vi "LDA_BSA_Comms_F600.vi"(2 "LDA Channels":T1[](array[typedef]) {"Sync Delay (s)" format="%.2g"; "Req Sampling Rate Hz" min=1.0; "Shifted mW" format="%.1g"; "Unshifted mW" format="%.1g"; "Centre Velocity (m/s)" format="%.2g"; "Velocity Range (m/s)" format="%.2g"; "Focal Length (mm)" format="%.1f"; "Beam Separation (mm)" format="%.1f"; "Optics Conversion Factor" format="%.3g"; "High voltage" min=0 max=2040 step=8; "Signal gain (dB)" min=0 max=30 step=1; "Min Velocity" format="%.2g"; "Max Velocity" format="%.2g"; "Wavelength (nm)" format="%.1f"}, 3 "BSACtrl.IBSA F600":refnum<k7>) -> (0 "error out":errorcluster, 1 "LDA Raw Data":cluster{dbl[][]}[](array[cluster]))   [LabVIEW 2021]
uses:
  LDA_Channel.ctl
  Globals/Meas_global.vi
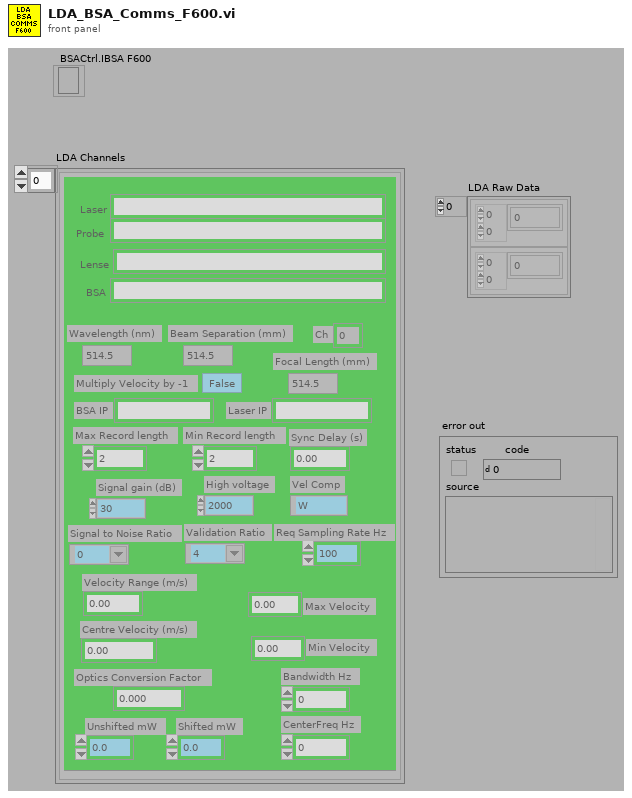
[diagram p1: front panel]
types:
  T1 = typedef "LDA_Channel.ctl" = cluster{"Wavelength (nm)":dbl, "Vel Comp":string, "Max Velocity":dbl, "Min Velocity":dbl, "Max Record length":u16, "Signal gain (dB)":i16, "High voltage":i16, "Optics Conversion Factor":dbl, "Min Record length":u16, "Multiply Velocity by -1":bool, "Signal to Noise Ratio":string, "Validation Ratio":string, "Probe":string, "Laser":string, "BSA":string, "Lense":string, "Beam Separation (mm)":dbl, "Focal Length (mm)":dbl, "COLOUR":u32, "BSA IP":string, "Velocity Range (m/s)":dbl, "Centre Velocity (m/s)":dbl, "Unshifted mW":dbl, "Shifted mW":dbl, "Bandwidth Hz":dbl, "Req Sampling Rate Hz":dbl, "Ch":i32, "CenterFreq Hz":dbl, "Laser IP":string, "Sync Delay (s)":dbl}
  T2 = typedef "Analysis_info_cluster.ctl" = cluster{"Colour":u32, "Inst type":T3, "Inst name":string, "Symbol":string, "Code name":string, "Extra Info":string, "Inst Array":T4, "Extra Titles":string[], "Extra Values":string[], "U":dbl, "u^2":dbl, "u^3":dbl, "u^4":dbl, "Skew_u":dbl, "Kurt_u":dbl, "Sd Error in Mean":dbl, "% u'/U":dbl, "X":dbl, "Y":dbl, "Z":dbl, "Timescale integral Estimate":dbl, "Sd Error in Variance":dbl, "Calib File":path, "Calib Constants":dbl[], "Output Position":bool, "Stats":enum16{"None", "Basic", "Full"}, "Av Sampling Rate":dbl, "Av No of Samples":dbl, "Total Meas Time (s)":dbl, "ADAM Ch Name":string, "Max value":dbl, "Min value":dbl, "Req Sample Rate Hz":dbl, "Sync Delay Time (s)":dbl, "Ch No":i16, "Device":string, "Use Latest Calib":bool, "Port":string, "Metadata Ch Names":string[], "Metadata Ch Values":string[], "Label":string}
  T3 = typedef "Inst_type.ctl" = enum16{"Raw voltage", "Raw with zero offsetting", "Propeller anemometer", "Pressure Transducer", "Pitot-static tube", "Hot wire", "Cross wire 1", "Cross wire 2", "Generic Linear", "Generic Polynomial", "Generic BackPoly", "Fast FID", "Thermocouple", "Cold wire", "Pulsed Wire", "LDA Vel", "LDA Tran time", "LDA Arr time", "Microphone"}
  T4 = typedef "Instrument_Array.ctl" = enum16{"PWA", "LDA", "Analogue"}
  T5 = typedef "Trigger_Mode.ctl" = enum16{"Free Running", "Start on Trigger", "Trigger Every Block", "Trigger Every Sample"}
  T6 = typedef "Rendezvous RefNum" = refnum<k1>
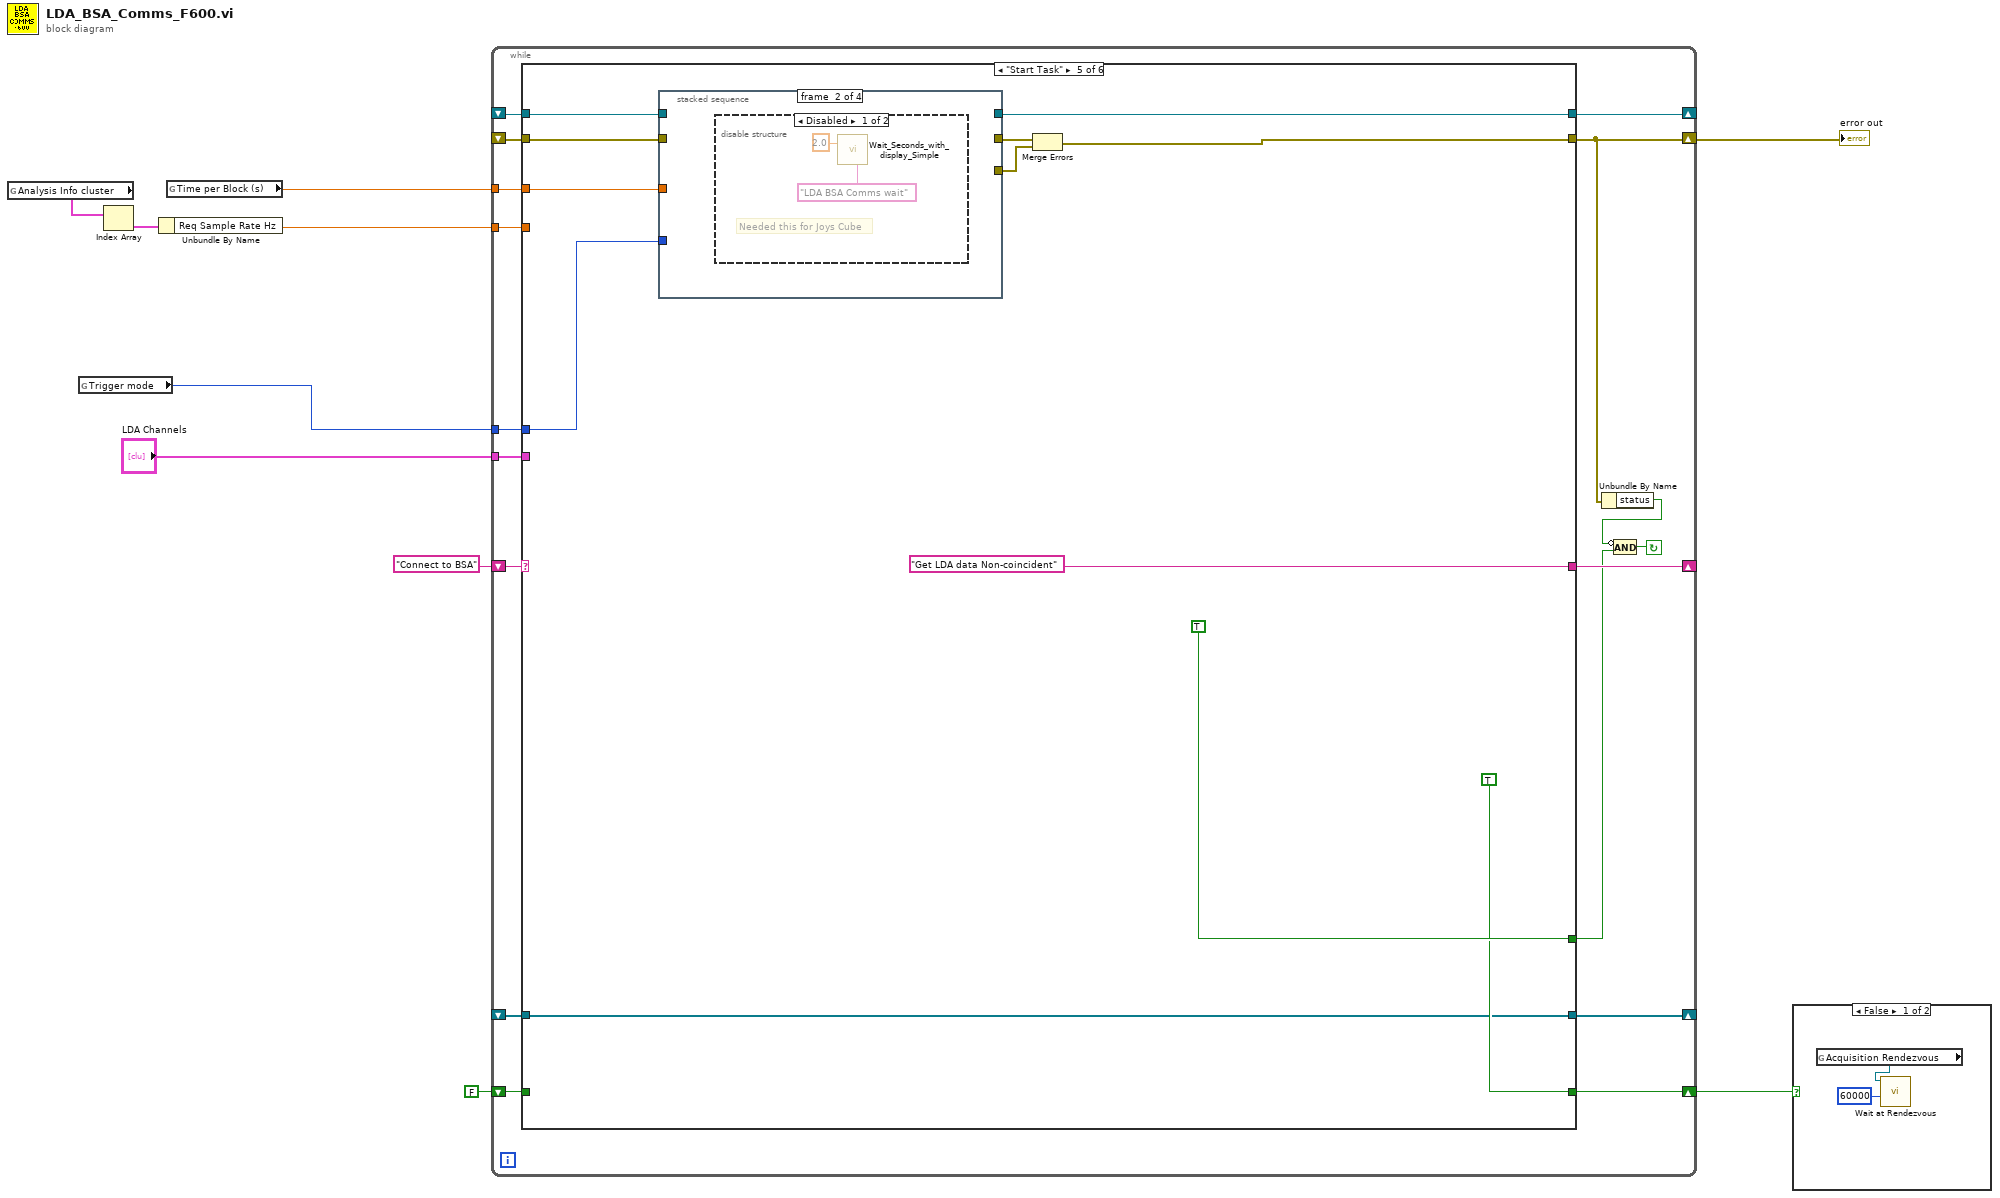
[diagram p0: block diagram]
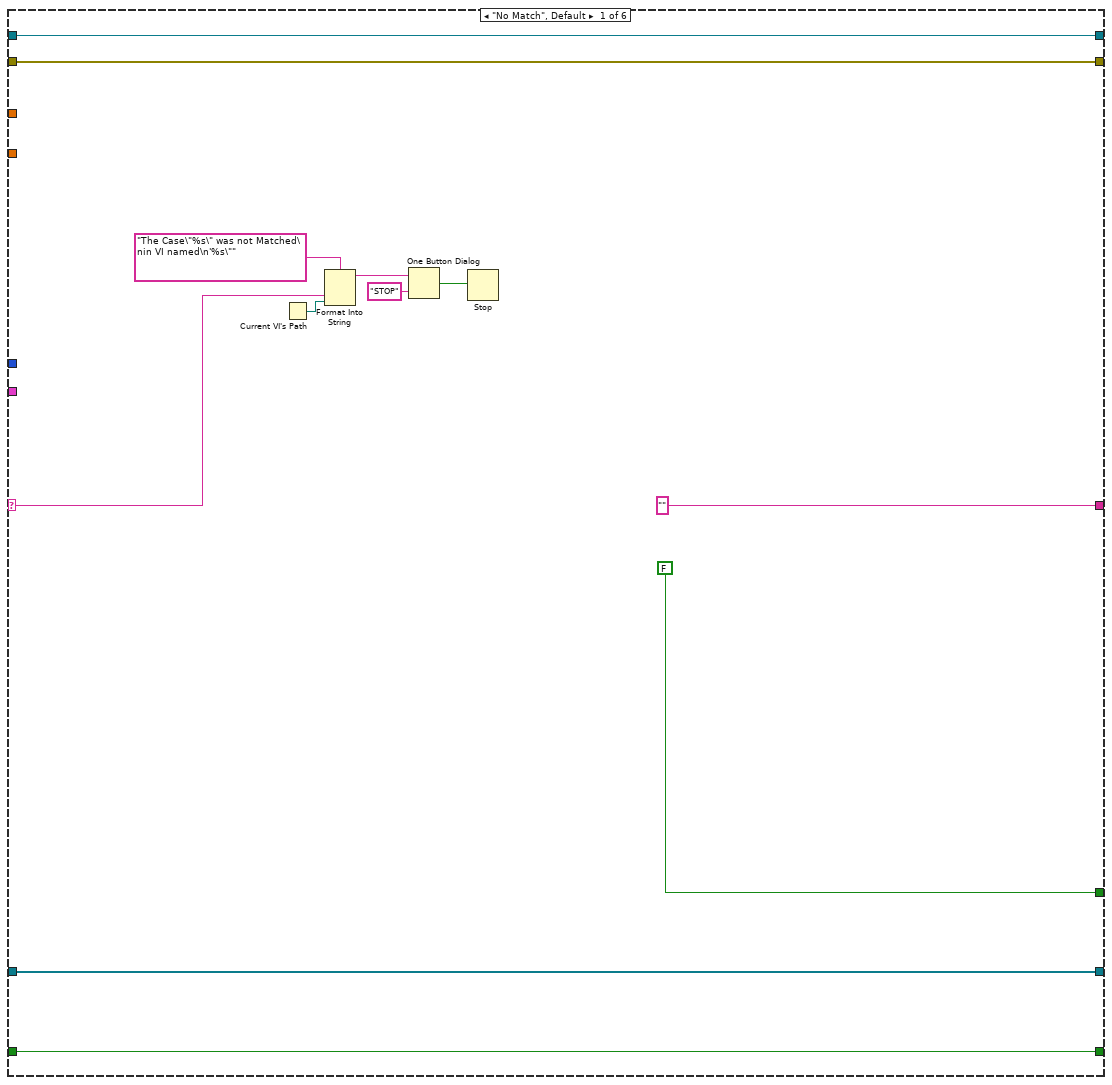
[diagram p2: hidden frame]
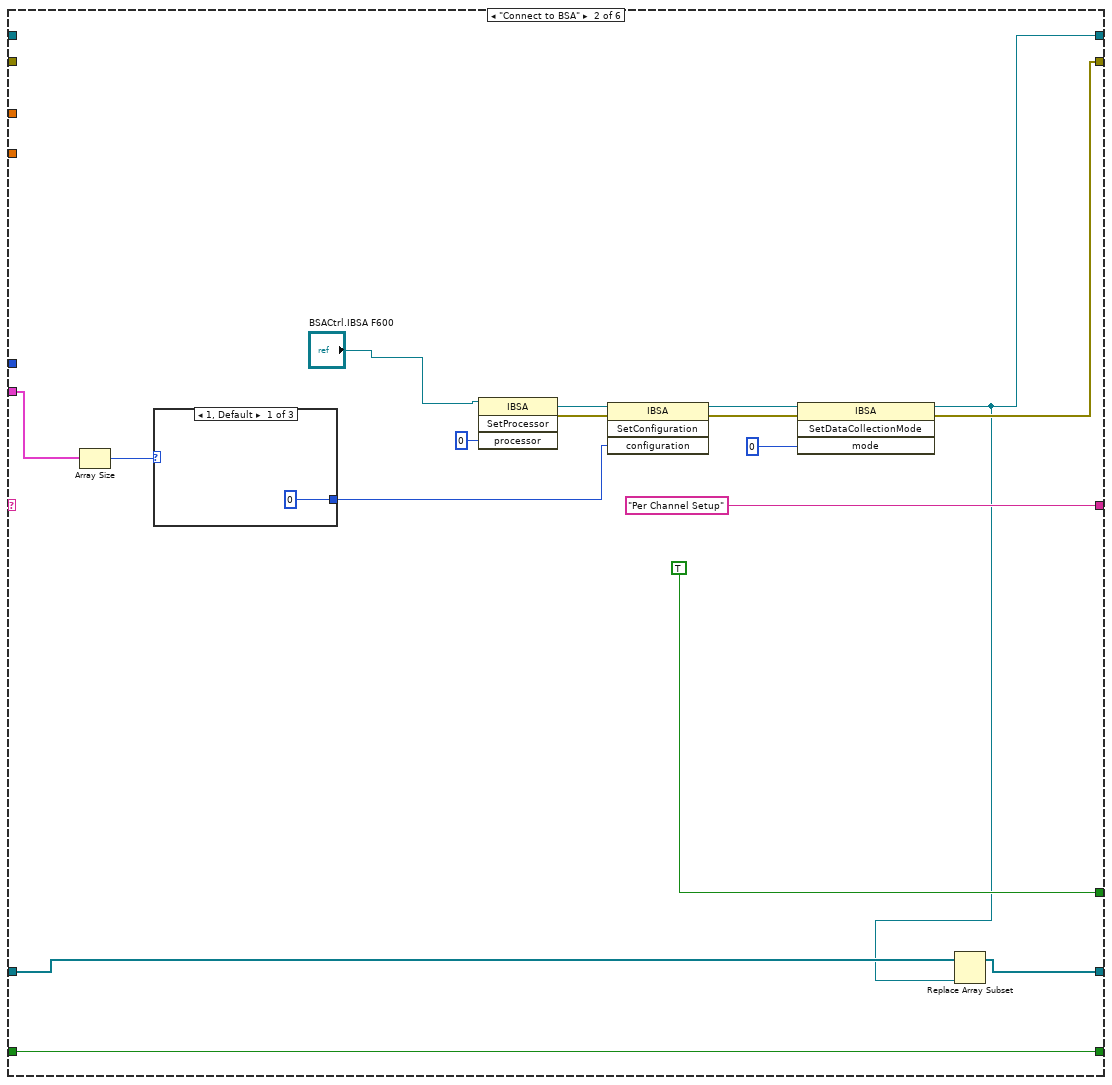
[diagram p3: hidden frame]
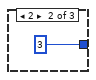
[diagram p4: hidden frame]
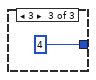
[diagram p5: hidden frame]
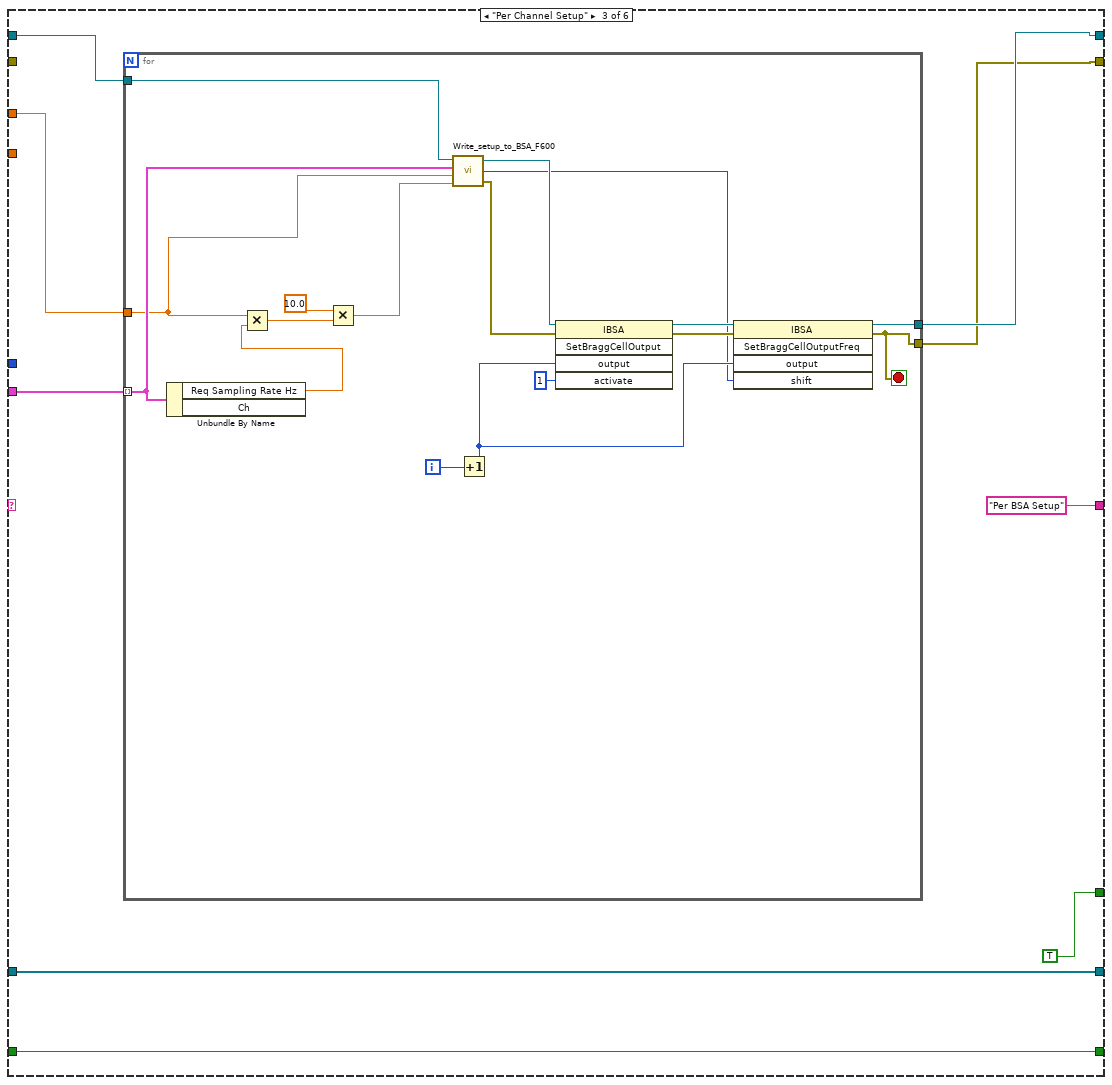
[diagram p6: hidden frame]
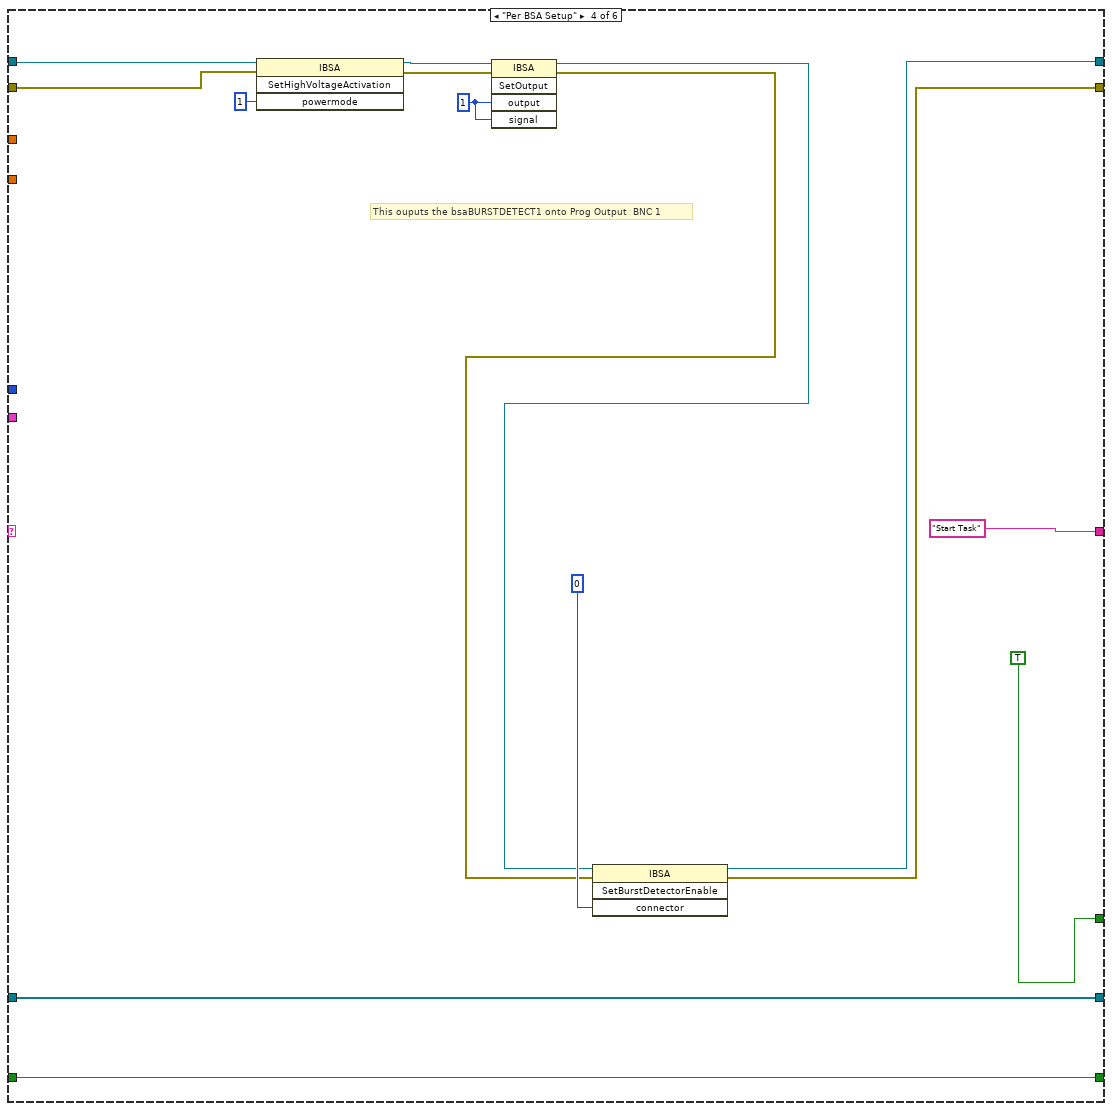
[diagram p7: hidden frame]
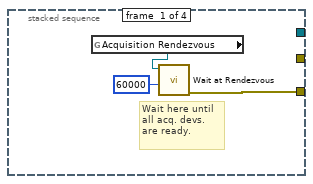
[diagram p8: hidden frame]
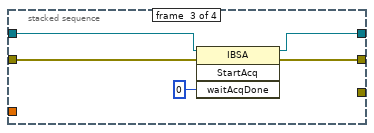
[diagram p10: hidden frame]
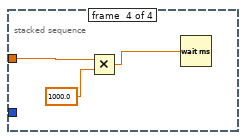
[diagram p11: hidden frame]
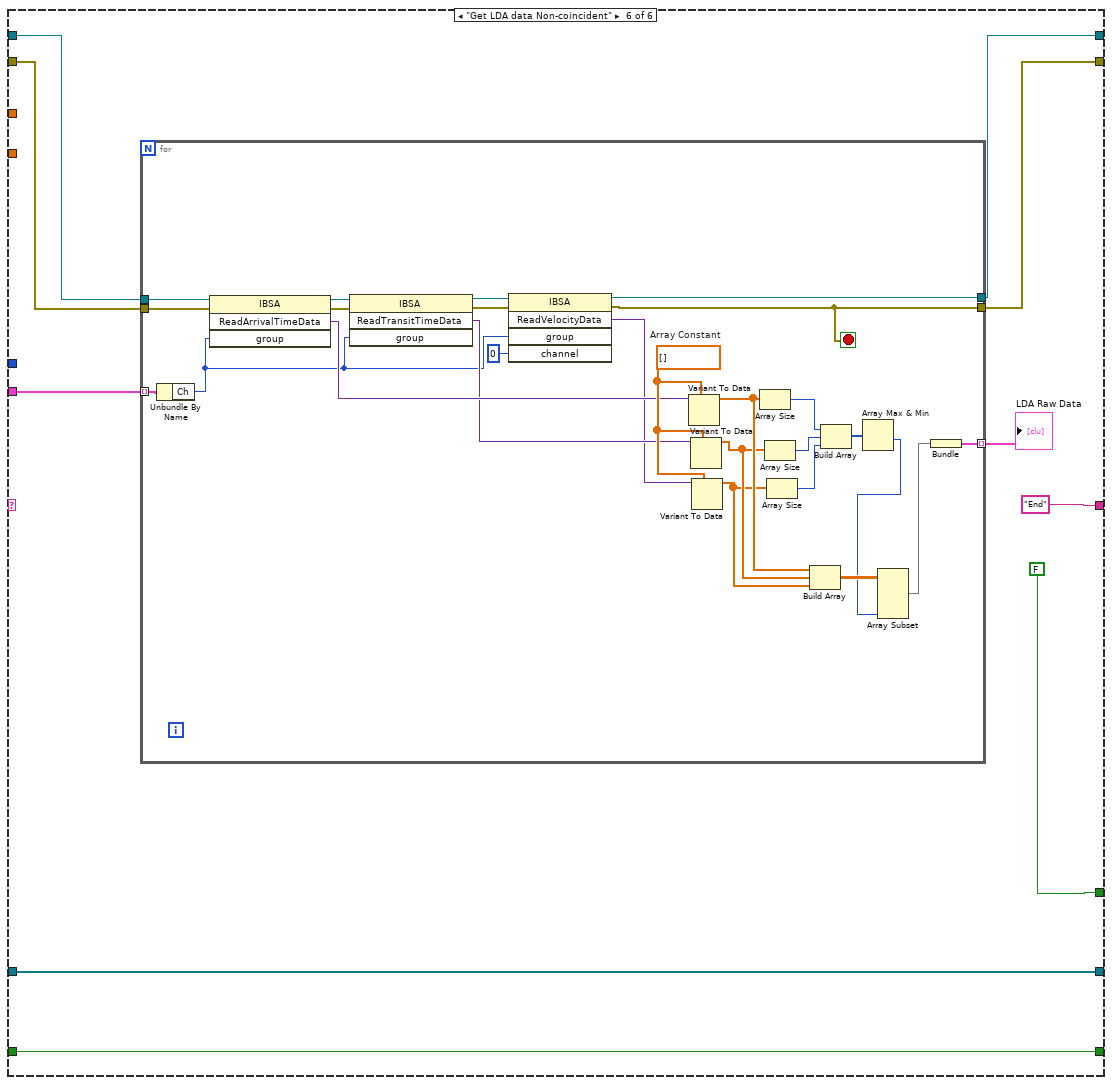
[diagram p12: hidden frame]
diagram:
  n1 = global read "Meas_global.vi" "Analysis Info cluster"() -> (w10:T2[])
  n2 = global read "Meas_global.vi" "Trigger mode"() -> (w6:T5)
  n3 = Index Array(array=w10) -> (element=w9:T2)  [unwired: 1 in]
  n4 = Unbundle By Name(w9) -> ("Req Sample Rate Hz"=w8:dbl)
  n5 = global read "Meas_global.vi" "Time per Block (s)"() -> (w7:dbl)
  n6 = while {
    shift-left: "Connect to BSA" -> [w26]
    shift-right: [w27] -> _
    shift-right: [w23] -> w1
    shift-left: _ -> [w16]
    tunnel: w8 -> [w25]
    shift-right: [w24] -> _
    shift-left: _ -> [w17]
    tunnel: w7 -> [w19]
    tunnel: w6 -> [w18]
    tunnel: "LDA Channels" -> [w15]
    shift-right: [w14] -> w5
    shift-left: FALSE -> [w13]
    shift-right: [w11] -> _
    shift-left: _ -> [w12]
    stop <- w21 continue-if-true
    n7 = case shown="\"Start Task\"" w26 {
      selector: w26 -> [w30 _ _ _ _ _]
      tunnel: [FALSE TRUE TRUE TRUE TRUE FALSE] -> w20
      tunnel: ["" "Per Channel Setup" "Per BSA Setup" "Start Task" "Get LDA data Non-coincident" "End"] -> w27
      tunnel: [w32 w48 w60 w95 w107 w131] -> w23
      tunnel: w16 -> [w32 _ _ w98 w105 w134]
      tunnel: w25 -> [_ _ _ _ _ _]
      tunnel: w17 -> [w31 _ w64 w99 w106 w135]
      tunnel: [w31 w45 w61 w96 w111 w127] -> w24
      tunnel: w19 -> [_ _ w67 _ w101 _]
      tunnel: w18 -> [_ _ _ _ w104 _]
      tunnel: w15 -> [_ w42 w65 _ _ w130]
      tunnel: [w29 w47 w63 w92 TRUE w129] -> w14
      tunnel: w13 -> [w29 w47 w63 w92 _ w129]
      tunnel: w12 -> [w28 w46 w62 w91 w102 w128]
      tunnel: [w28 w44 w62 w91 w102 w128] -> w11
      frame "No Match", Default {
        n8 = Current VI's Path() -> (path=w34:path)
        n9 = Format Into String(format string="The Case\"%s\" was not Matched\nin VI named\n'%s\"" ("Format String"), w30, w34) -> (resulting string=w37:string)  [unwired: 2 in, 1 out]
        n10 = One Button Dialog(message=w37, button name ("OK")="STOP") -> (true=w35:bool)
        n11 = Stop(stop? (T)=w35) -> ()
      }
      frame "Connect to BSA" {
        n12 = Array Size(array=w42) -> (size(s)=w41:i32)
        n13 = case shown="1, Default" w41 {
          tunnel: [0 ("configuration") 3 ("configuration") 4 ("configuration")] -> w40
          frame 1, Default {
          }
          frame 2 {
          }
          frame 3 {
          }
        }
        n14 = invoke class="IBSA" method="SetProcessor"(reference="BSACtrl.IBSA F600", "processor"=0) -> (reference out=w53:refnum<k7>, error out=w52:errorcluster)  [unwired: 2 in, 2 out]
        n15 = invoke class="IBSA" method="SetConfiguration"(reference=w53, error in=w52, "configuration"=w40) -> (reference out=w51:refnum<k7>, error out=w50:errorcluster)  [unwired: 1 in, 2 out]
        n16 = invoke class="IBSA" method="SetDataCollectionMode"(reference=w51, error in=w50, "mode"=0) -> (reference out=w45:refnum<k7>, error out=w48:errorcluster)  [unwired: 1 in, 2 out]
        n17 = Replace Array Subset(array=w46, new element=w45) -> (w44:refnum<k7>[])  [unwired: 1 in]
      }
      frame "Per Channel Setup" {
        n18 = for {
          tunnel: w67 -> [w80]
          tunnel: w65 -> [w81] mode=indexing
          tunnel: w64 -> [w82]
          tunnel: [w70] -> w61
          tunnel: [w69] -> w60
          i -> [w72]
          stop <- w69 stop-if-true
          n19 = Unbundle By Name(w81) -> ("Req Sampling Rate Hz"=w83:dbl)  [unwired: 1 out]
          n20 = Multiply(x=w80, y=w83) -> (x*y=w84:dbl)
          n21 = Multiply(x=10.0 ("y"), y=w84) -> (x*y=w79:dbl)
          n22 = call "Write_setup_to_BSA_F600.vi"("No Of Samples"=w79, "Time (s)"=w80, "BSA Setup In"=w81, "BSACtrl.IBSA F600"=w82) -> ("error out"=w75:errorcluster, "Frequecy Shift (MHz)"=w71:i32, "BSACtrl.IBSA F600 Out"=w74:refnum<k7>)
          n23 = Increment(x=w72) -> (x+1=w73:i32)
          n24 = invoke class="IBSA" method="SetBraggCellOutput"(reference=w74, error in=w75, "output"=w73, "activate"=1) -> (reference out=w77:refnum<k7>, error out=w76:errorcluster)  [unwired: 1 in, 3 out]
          n25 = invoke class="IBSA" method="SetBraggCellOutputFreq"(reference=w77, error in=w76, "output"=w73, "shift"=w71) -> (reference out=w70:refnum<k7>, error out=w69:errorcluster)  [unwired: 1 in, 3 out]
        }
      }
      frame "Per BSA Setup" {
        w86 = 1 ("output")
        # "This ouputs the bsaBURSTDETECT1 onto Prog Output  BNC 1"
        n26 = invoke class="IBSA" method="SetHighVoltageActivation"(reference=w99, error in=w98, "powermode"=1) -> (reference out=w90:refnum<k7>, error out=w89:errorcluster)  [unwired: 1 in, 2 out]
        n27 = invoke class="IBSA" method="SetOutput"(reference=w90, error in=w89, "output"=w86, "signal"=w86) -> (reference out=w88:refnum<k7>, error out=w87:errorcluster)  [unwired: 1 in, 3 out]
        n28 = invoke class="IBSA" method="SetBurstDetectorEnable"(reference=w88, error in=w87, "connector"=0) -> (reference out=w96:refnum<k7>, error out=w95:errorcluster)  [unwired: 1 in, 2 out]
      }
      frame "Start Task" {
        n29 = stacked-sequence {
          tunnel: [_ _ w119 _] -> w109
          tunnel: w106 -> [_ _ w120 _]
          tunnel: [_ _ w118 _] -> w111
          tunnel: w105 -> [_ _ w121 _]
          tunnel: [w114 _ _ _] -> w108
          tunnel: w104 -> [_ _ _ _]
          tunnel: w101 -> [_ _ _ w125]
          frame #0 {
            # "Wait here until all acq. devs. are ready."
            n30 = global read "Meas_global.vi" "Acquisition Rendezvous"() -> (w115:T6)
            n31 = call <vilib>:"Wait at Rendezvous.vi"("ms timeout (-1)"=60000, "rendezvous"=w115) -> ("error out"=w114:errorcluster)  [unwired: 3 in, 2 out]
          }
          frame #1 {
            n32 = disable-structure shown="Disabled" {
              frame Disabled {
                # "Needed this for Joys Cube"
                n33 = call "Wait_Seconds_with_display_Simple.vi"("Message"="LDA BSA Comms wait", "Seconds to wait"=2.0) -> ()  [unwired: 1 in, 1 out]
              }
              frame Enabled {
              }
            }
          }
          frame #2 {
            n34 = invoke class="IBSA" method="StartAcq"(reference=w120, error in=w121, "waitAcqDone"=0) -> (reference out=w118:refnum<k7>, error out=w119:errorcluster)  [unwired: 1 in, 2 out]
          }
          frame #3 {
            n35 = Multiply(x=w125, y=1000.0) -> (x*y=w123:dbl)
            n36 = Wait (ms)(milliseconds to wait=w123) -> ()  [unwired: 1 out]
          }
        }
        n37 = Merge Errors(w109, w108) -> (w107:errorcluster)
      }
      frame "Get LDA data Non-coincident" {
        n38 = for {
          tunnel: w135 -> [w153]
          tunnel: w134 -> [w152]
          tunnel: [w151] -> w126 mode=indexing
          tunnel: [w150] -> w127
          tunnel: [w149] -> w131
          tunnel: w130 -> [w148] mode=indexing
          stop <- w149 stop-if-true
          w157 = dbl[] []  # Array Constant
          n39 = Unbundle By Name(w148) -> ("Ch"=w147:i32)
          n40 = invoke class="IBSA" method="ReadArrivalTimeData"(reference=w153, error in=w152, "group"=w147) -> (reference out=w161:refnum<k7>, error out=w160:errorcluster, "ReadArrivalTimeData"=w156:variant)  [unwired: 1 in, 1 out]
          n41 = invoke class="IBSA" method="ReadTransitTimeData"(reference=w161, error in=w160, "group"=w147) -> (reference out=w159:refnum<k7>, error out=w158:errorcluster, "ReadTransitTimeData"=w155:variant)  [unwired: 1 in, 1 out]
          n42 = invoke class="IBSA" method="ReadVelocityData"(reference=w159, error in=w158, "group"=w147, "channel"=0) -> (reference out=w150:refnum<k7>, error out=w149:errorcluster, "ReadVelocityData"=w154:variant)  [unwired: 1 in, 2 out]
          n43 = Variant To Data(type=w157, Variant=w156) -> (data=w141:dbl[])  [unwired: 1 in, 1 out]
          n44 = Variant To Data(type=w157, Variant=w155) -> (data=w140:dbl[])  [unwired: 1 in, 1 out]
          n45 = Variant To Data(type=w157, Variant=w154) -> (data=w139:dbl[])  [unwired: 1 in, 1 out]
          n46 = Array Size(array=w141) -> (size(s)=w143:i32)
          n47 = Array Size(array=w140) -> (size(s)=w144:i32)
          n48 = Array Size(array=w139) -> (size(s)=w145:i32)
          n49 = Build Array(w141, w140, w139) -> (w138:dbl[][])
          n50 = Build Array(w143, w144, w145) -> (w142:i32[])
          n51 = Array Max & Min(array=w142) -> (min value=w137:i32)  [unwired: 3 out]
          n52 = Array Subset(array=w138, length (col)=w137) -> (w136:dbl[][])  [unwired: 3 in]
          n53 = Bundle(w136) -> (w151:cluster{dbl[][]})  [unwired: 1 in]
        }
        "LDA Raw Data" <- w126
      }
    }
    n54 = Unbundle By Name(w23) -> ("status"=w22:bool)
    n55 = Compound Arithmetic op=AND(invert w22, w20) -> (w21:bool)
  }
  "error out" <- w1
  n56 = case shown="False" w5 {
    frame False {
      n57 = global read "Meas_global.vi" "Acquisition Rendezvous"() -> (w162:T6)
      n58 = call <vilib>:"Wait at Rendezvous.vi"("ms timeout (-1)"=60000, "rendezvous"=w162) -> ()  [unwired: 3 in, 3 out]
    }
    frame True {
    }
  }
